vi "calc centroid predict and correct_TBDEL.vi"(0 "Queue in":refnum<queue>, 1 "Session Out":T3, 2 "Save":T4, 5 "# Images in Burst":i32, 7 "Python session":refnum<k35>, 9 "Enable Python":bool, 11 "error in (no error)":errorcluster, 12 "module path":path, 13 "reference":refnum<k24>, 14 "PIezo Voltages":dbl[](array[numeric])) -> (6 "tdms ref out":refnum<k34>, 8 "mean":dbl format="%0.2f", 15 "error out":errorcluster)   [LabVIEW 2020]
uses:
  <vilib>/vision/Image Controls.llb/IMAQ Image.ctl
  <vilib>/userDefined/High Color/IMAQdx.ctl
  threshold ctl.ctl
  tdms options.ctl
  C:/GEECS/Developers Version/source/Device Drivers/Point Grey Camera/fast camera acquisition/Thorlabs.MotionControl.Controls.dll
  Thorlabs.MotionControl.Controls.dll
  C:/GEECS/Developers Version/source/Device Drivers/Point Grey Camera/fast camera acquisition/Thorlabs.MotionControl.KCube.PiezoCLI.dll
  Thorlabs.MotionControl.KCube.PiezoCLI.dll
  <vilib>/Analysis/baseanly.llb/Mean (DBL).vi
  <vilib>/Utility/High Resolution Relative Seconds.vi
  <vilib>/vision/driver/NI_Vision_Acquisition_Software.lvlib
  <vilib>/Analysis/NI_AALBase.lvlib
panel:
  in  "Tab Control":enum32{"Main", "Internal"}(tab)
  in  "Threshold":T1={"Use threshold fraction"=TRUE, "threshold fraction"=0.8, "Threshold Range"={"Lower value"=128.0, "Upper value"=255.0}}
  out "Waveform Chart":T2(graph)
  out "Images Processed":u32
  out "# elements in queue":i32
  out "Current Buffer Number":u32
  out "processed in burst":u32
  out "image processing time (ms)":dbl caption="loop time (ms)"
  out "Avg Error (px)":dbl format="%0.2f"
  out "Std measured (px)":dbl format="%0.2f"
  out "Std diff (px)":dbl format="%0.2f"
  out "loop time (us)":dbl caption="loop time (us) not in use"
  out "Avg loop time (ms)":dbl
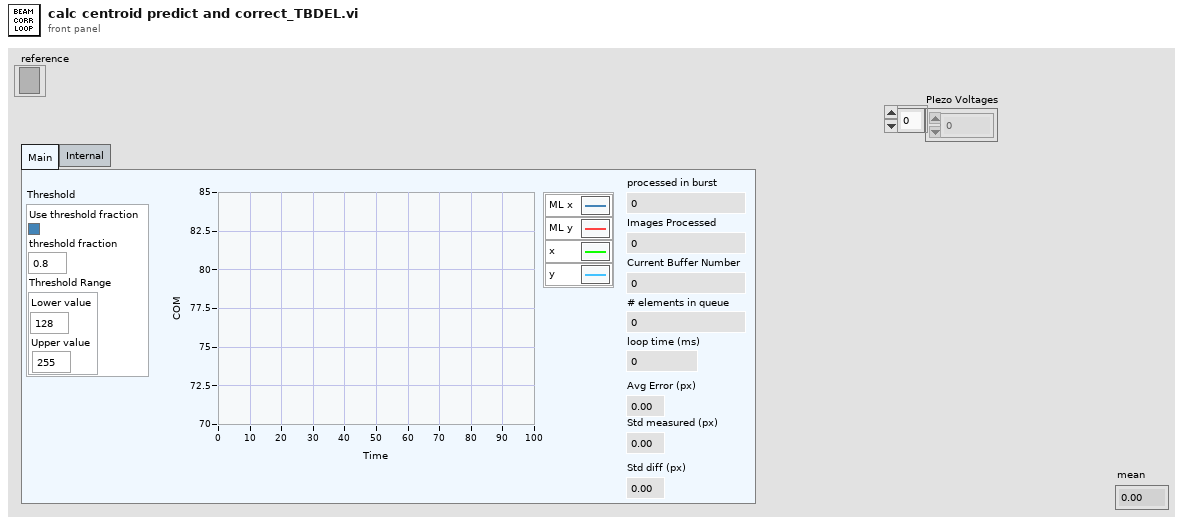
[diagram p1: front panel]
types:
  T1 = typedef "threshold ctl.ctl" = cluster{"Use threshold fraction":bool, "threshold fraction":sgl, "Threshold Range":cluster{"Lower value":sgl, "Upper value":sgl}}
  T2 = cluster{"X Centroid":dbl, "X Centroid":dbl, "X Centroid":sgl, "Y Centroid":sgl}
  T3 = typedef "IMAQdx.ctl" = refnum<k21>
  T4 = typedef "tdms options.ctl" = cluster{"save":bool, "tdms filename prefix":string, "tdms folder path":path}
  T5 = cluster{"X Centroid":dbl, "X Centroid":dbl, "X Centroid":sgl, "Y Centroid":sgl}[]
  T6 = typedef "IMAQ Image.ctl" = refnum<image>
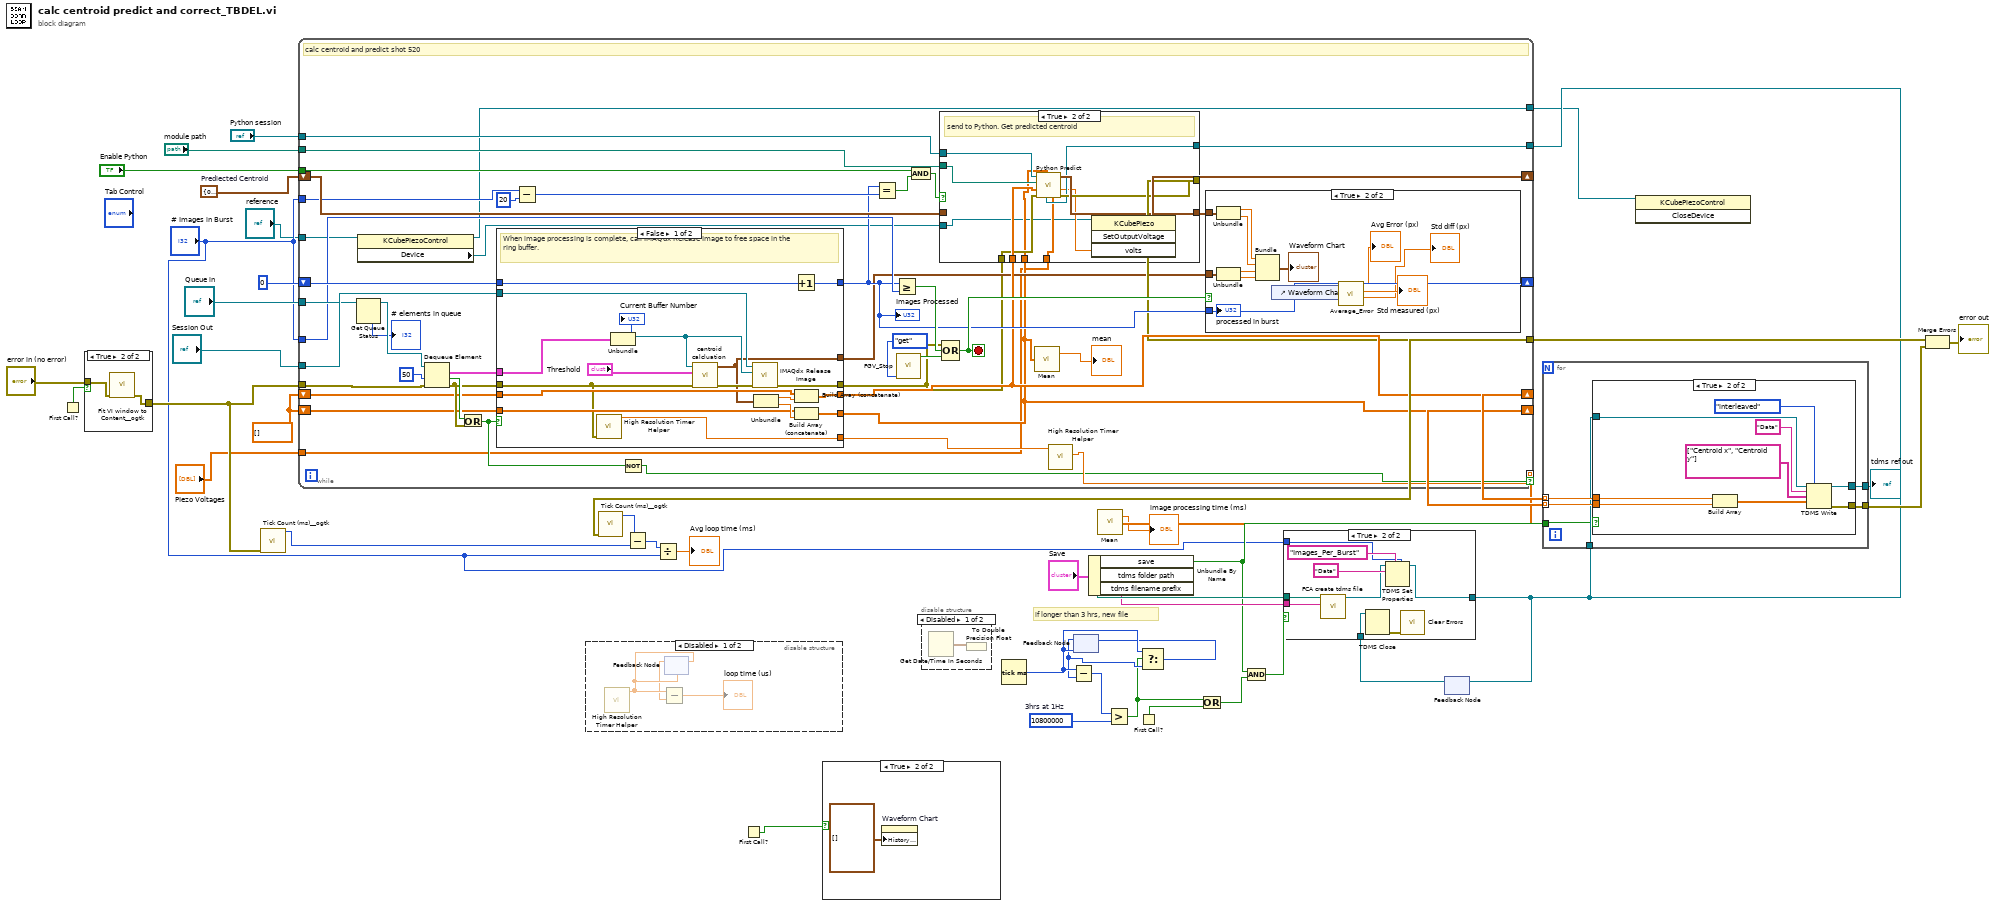
[diagram p0: block diagram]
diagram:
  w23 = i64 10800000  # 3hrs at 1Hz
  w42 = cluster{"X Centroid":sgl, "Y Centroid":sgl} {"X Centroid"=0.0, "Y Centroid"=0.0}  # Prediected Centroid
  w41 = sgl[] []
  # "if longer than 3 hrs, new file"
  n1 = First Call?() -> (First Call?: T/F=w27:bool)
  n2 = case shown="True" w27 {
    tunnel: "error in (no error)" -> [w44 w46]
    tunnel: [w44 w45] -> w28
    frame False {
    }
    frame True {
      n3 = call <userlib>:"Fit VI window to Content__ogtk.vi"("error in (no error)"=w46) -> ("error out"=w45:errorcluster)  [unwired: 5 in, 1 out]
    }
  }
  n4 = call <userlib>:"Tick Count (ms)__ogtk.vi"("error in (no error)"=w28) -> ("millisecond timer value"=w32:u32)  [unwired: 9 in, 1 out]
  n5 = disable-structure shown="Disabled" {
    frame Disabled {
      n6 = call "High Resolution Timer Helper.vi"() -> ("Current Time"=w49:dbl)  [unwired: 9 in, 2 out]
      n7 = feedback #1(w49) -> (w47:dbl)
      n8 = Subtract(x=w49, y=w47) -> (x-y=→"loop time (us)":dbl)
      n9 = feedback-in #1(w49) -> ()
    }
    frame Enabled {
    }
  }
  n10 = First Call?() -> (First Call?: T/F=w6:bool)
  n11 = case shown="True" w6 {
    frame False {
    }
    frame True {
      n12 = property on="Waveform Chart" class="WFChart (strict)"("History Data"=T5 []) -> ()  [unwired: 2 in, 2 out]
    }
  }
  n13 = disable-structure shown="Disabled" {
    frame Disabled {
      n14 = Get Date/Time In Seconds() -> (seconds since 1Jan1904=w51:timestamp)
      n15 = To Double Precision Float(number=w51) -> ()  [unwired: 1 out]
    }
    frame Enabled {
    }
  }
  n16 = Tick Count (ms)() -> (millisecond timer value=w21:u32)
  n17 = feedback #2(w21) -> (w19:u32)
  n18 = Subtract(x=w21, y=w19) -> (x-y=w22:u32)
  n19 = Unbundle By Name("Save") -> ("save"=w14:bool, "tdms folder path"=w26:path, "tdms filename prefix"=w25:string)
  n20 = Greater?(x=w22, y=w23) -> (0:w12:bool)
  n21 = First Call?() -> (First Call?: T/F=w11:bool)
  n22 = Select(t=w21, s=w12, f=w19) -> (s? t:f=w20:u32)
  n23 = feedback-in #2(w20) -> ()
  n24 = Or(x=w12, y=w11) -> (x .or. y?=w10:bool)
  n25 = And(x=w14, y=w10) -> (x .and. y?=w18:bool)
  n26 = feedback #3() -> (w17:refnum<k34>)  [unwired: 1 in]
  n27 = case shown="True" w18 {
    tunnel: [w52 w54] -> w5
    tunnel: w25 -> [_ w61]
    tunnel: w26 -> [_ w60]
    tunnel: w17 -> [w52 w58]
    tunnel: "# Images in Burst" -> [_ w53]
    frame False {
    }
    frame True {
      n28 = call "FCA create tdms file.vi"("Filename prefix"=w61, "Folder path"=w60) -> ("Refnum out"=w55:refnum<k34>)  [unwired: 8 in, 1 out]
      n29 = TDMS Close(11:w58) -> (0:w59:errorcluster)  [unwired: 1 in, 1 out]
      n30 = TDMS Set Properties(5:w53, 7:"Images_Per_Burst", 10:"Data" ("group name in (Untitled)"), 11:w55) -> (3:w54:refnum<k34>)  [unwired: 2 in, 3 out]
      n31 = call <vilib>:"Clear Errors.vi"("error in (no error)"=w59) -> ()  [unwired: 5 in, 2 out]
    }
  }
  n32 = while {
    tunnel: [w76] -> w34
    tunnel: "Queue in" -> [w93]
    tunnel: "Session Out" -> [w102]
    shift-right: [w83] -> _
    shift-left: u32 0 -> [w101]
    tunnel: w28 -> [w72]
    shift-right: [w82] -> w16
    shift-left: w41 -> [w97]
    shift-right: [w66] -> w15
    shift-left: w41 -> [w96]
    shift-right: [w94] -> _
    shift-left: w42 -> [w95]
    tunnel: "# Images in Burst" -> [w90]
    tunnel: "# Images in Burst" -> [w86]
    tunnel: "Python session" -> [w81]
    tunnel: "Enable Python" -> [w79]
    tunnel: "module path" -> [w77]
    tunnel: [w73] -> w8 mode=indexing if=w69
    tunnel: w5 -> [w68]
    tunnel: "reference" -> [w65]
    tunnel: "PIezo Voltages" -> [w63]
    tunnel: [w64] -> w1
    stop <- w98 stop-if-true
    # "calc centroid and predict shot 520"
    n33 = Get Queue Status(queue=w93) -> (queue out=w92:refnum<queue>, # elements in queue=→"# elements in queue":i32)  [unwired: 2 in, 6 out]
    n34 = property class="KCubePiezoControl"(reference=w65) -> (reference out=w64:refnum<k24>, "Device"=w62:refnum<k24>)  [unwired: 1 in, 1 out]
    n35 = Dequeue Element(queue=w92, timeout in ms (-1)=50 ("timeout in ms"), error in (no error)=w72) -> (element=w103:cluster{"Image Out":T6, "Buffer Number Out":u32}, timed out?=w100:bool, error out=w99:errorcluster)  [unwired: 1 out]
    n36 = Or(x=w100, y=w99) -> (x .or. y?=w70:bool)
    n37 = case shown="False" w70 {
      tunnel: w99 -> [w130 w151]
      tunnel: w103 -> [w147 _]
      tunnel: [w146 w151] -> w74
      tunnel: w102 -> [w145 _]
      tunnel: w101 -> [w143 w150]
      tunnel: [w142 w150] -> w83
      tunnel: w97 -> [w141 w149]
      tunnel: [w139 w149] -> w82
      tunnel: [w137 w148] -> w66
      tunnel: w96 -> [w136 w148]
      tunnel: [w133 _] -> w75
      tunnel: [w131 _] -> w71
      frame False {
        # "When image processing is complete, call IMAQdx Release Image to free space in the ring buffer."
        n38 = call "High Resolution Timer Helper.vi"("error in (no error)"=w130) -> ("Current Time"=w131:dbl)  [unwired: 8 in, 2 out]
        n39 = Unbundle(w147) -> ("Image Out"=w135:T6, "Buffer Number Out"=→"Current Buffer Number":u32)
        n40 = call "centroid calcluation.vi"("error in (no error)"=w130, "Threshold"="Threshold", "Refnum in"=w135) -> ("error out"=w134:errorcluster, "Centroid"=w133:cluster{"X Centroid":sgl, "Y Centroid":sgl})  [unwired: 6 in, 1 out]
        n41 = call <vilib>:"IMAQdx Release Image.vi"("error in"=w134, "Image"=w135, "Session In"=w145) -> ("error out"=w146:errorcluster)  [unwired: 7 in, 1 out]
        n42 = Unbundle(w133) -> ("X Centroid"=w140:sgl, "Y Centroid"=w138:sgl)
        n43 = Increment(x=w143) -> (x+1=w142:u32)
        n44 = Build Array (concatenate)(w141, w140) -> (w139:sgl[])
        n45 = Build Array (concatenate)(w136, w138) -> (w137:sgl[])
      }
      frame True {
        # "Empty queue or error.\nNothing to process."
      }
    }
    "Images Processed" <- w83
    n46 = Subtract(x=w90, y=20) -> (x-y=w88:i32)
    n47 = Not(x=w70) -> (.not. x?=w69:bool)
    n48 = Equal?(x=w83, y=w88) -> (x = y?=w80:bool)
    n49 = Greater Or Equal?(x=w83, y=w86) -> (x >= y?=w87:bool)
    n50 = call "FGV_Stop.vi"("command"=enum16{"set", "get"}."get") -> ("stop"=w84:bool)  [unwired: 10 in]
    n51 = And(x=w79, y=w80) -> (x .and. y?=w78:bool)
    n52 = case shown="True" w78 {
      tunnel: w95 -> [w106 _]
      tunnel: [w106 w115] -> w94
      tunnel: w82 -> [_ w114]
      tunnel: w66 -> [_ w110]
      tunnel: w81 -> [_ w117]
      tunnel: w77 -> [_ w116]
      tunnel: w74 -> [w105 w112]
      tunnel: [w105 w113] -> w76
      tunnel: w68 -> [_ w111]
      tunnel: w63 -> [_ w108]
      tunnel: w62 -> [_ w107]
      frame False {
      }
      frame True {
        # "send to Python. Get predicted centroid"
        n53 = call "Python Predict.vi"("Piezo_Volts"=w108, "tdms file"=w111, "Array"=w110, "error in (no error)"=w112, "Array 2"=w114, "module path"=w116, "Refnum in"=w117) -> ("error out"=w113:errorcluster, "piezo volt Pred"=w109:dbl, "Cluster"=w115:cluster{"X Centroid":dbl, "X Centroid":dbl})  [unwired: 2 in]
        n54 = invoke class="KCubePiezo" method="SetOutputVoltage"(reference=w107, "volts"=w109) -> ()  [unwired: 2 in, 4 out]
      }
    }
    n55 = Compound Arithmetic op=OR(w74, w87, w84) -> (w98:bool)
    n56 = call-poly <vilib>:"Mean.vi"("X"=w66) -> ("mean"=→"mean":dbl)  [unwired: 1 out]
    n57 = call "High Resolution Timer Helper.vi"("Previous Time"=w71) -> ("Time Difference (ms)"=w73:dbl)  [unwired: 8 in, 2 out]
    n58 = case shown="True" w98 {
      tunnel: w94 -> [_ w128]
      tunnel: w75 -> [_ w129]
      tunnel: w83 -> [_ w122]
      frame False {
      }
      frame True {
        n59 = Unbundle(w128) -> ("X Centroid"=w127:dbl, "X Centroid"=w126:dbl)
        n60 = Unbundle(w129) -> ("X Centroid"=w125:sgl, "Y Centroid"=w124:sgl)
        n61 = Bundle("X Centroid"=w127, "X Centroid"=w126, "X Centroid"=w125, "Y Centroid"=w124) -> (→"Waveform Chart":T2)  [unwired: 1 in]
        n62 = control-ref of="Waveform Chart"() -> (w121:refnum<vi>)
        n63 = call "Average_Error.vi"("WaveformChart in"=w121) -> ("Std deviation diff"=→"Std diff (px)":dbl, "Std measured (px)"=→"Std measured (px)":dbl, "Avg Error (px)"=→"Avg Error (px)":dbl)  [unwired: 8 in]
        "processed in burst" <- w122
      }
    }
  }
  n64 = call <userlib>:"Tick Count (ms)__ogtk.vi"("error in (no error)"=w34) -> ("millisecond timer value"=w33:u32)  [unwired: 9 in, 1 out]
  n65 = Subtract(x=w33, y=w32) -> (x-y=w31:u32)
  n66 = Divide(x=w31, y="# Images in Burst") -> (x/y=→"Avg loop time (ms)":dbl)
  n67 = call-poly <vilib>:"Mean.vi"("X"=w8) -> ("mean"=→"image processing time (ms)":dbl)  [unwired: 1 out]
  n68 = feedback-in #3(w5) -> ()
  n69 = for {
    tunnel: w16 -> [w157] mode=indexing
    tunnel: w15 -> [w156] mode=indexing
    tunnel: w5 -> [w155]
    tunnel: w14 -> [w154]
    tunnel: [w153] -> w13
    tunnel: [w152] -> w9
    n70 = case shown="True" w154 {
      tunnel: w155 -> [w158 w163]
      tunnel: [w158 w162] -> w153
      tunnel: w157 -> [_ w161]
      tunnel: w156 -> [_ w160]
      tunnel: [_ w159] -> w152
      frame False {
      }
      frame True {
        n71 = Build Array(w161, w160) -> (w165:sgl[])
        n72 = TDMS Write(0:w163, 1:enum16{"decimated", "interleaved"}."interleaved" ("data layout (0:decimated)"), 5:"Data" ("group name in (Untitled)"), 7:string[] ["Centroid x", "Centroid y"] ("channel name(s) in (Untitled)"), 9:w165) -> (4:w162:refnum<k34>, 15:w159:errorcluster)  [unwired: 1 in, 2 out]
      }
    }
  }
  "tdms ref out" <- w13
  n73 = invoke class="KCubePiezoControl" method="CloseDevice"(reference=w1) -> ()  [unwired: 2 in, 3 out]
  n74 = Merge Errors(w34, w9) -> (→"error out":errorcluster)
